vi "Lift_State_Machine.vi"() -> ()   [LabVIEW 2016]
doc: "The state machine for the Lift System.\nDrives the lift forward, then upward, then back, then down to its origin."
uses:
  <vilib>/myRIO/Instrument Drivers/Onboard IO/AI/typedefs/AI Reference.ctl
  <vilib>/myRIO/Common/Instrument Driver Framework/Utilities/typedefs/myRIO Generic Hardware Reference.ctl
  <vilib>/myRIO/Common/Instrument Driver Framework/Utilities/typedefs/Hardware Version Enum.ctl
  <vilib>/myRIO/Common/Instrument Driver Framework/Utilities/typedefs/myRIO v1.0 Reference.ctl
  <vilib>/myRIO/Common/Instrument Driver Framework/Utilities/typedefs/Generic FPGA Reference.ctl
  <vilib>/myRIO/Common/Instrument Driver Framework/myRIO v1.0/AI/typedefs/AI Channels List.ctl
  <vilib>/myRIO/Common/Instrument Driver Framework/myRIO v1.0/AI/typedefs/AI Channels Enum.ctl
  <vilib>/myRIO/Common/Instrument Driver Framework/Utilities/typedefs/Analog Scaling Constants List.ctl
  <vilib>/myRIO/Common/Instrument Driver Framework/Utilities/typedefs/Analog Scaling Constants.ctl
  <vilib>/userdefined/High Color/nirio_resource_hc.ctl
  <vilib>/myRIO/Instrument Drivers/Onboard IO/DIO/typedefs/DIO Reference.ctl
  <vilib>/myRIO/Common/Instrument Driver Framework/myRIO v1.0/DIO/typedefs/DIO Channels List.ctl
  <vilib>/myRIO/Common/Instrument Driver Framework/myRIO v1.0/DIO/typedefs/DIO Channels Enum.ctl
  <vilib>/myRIO/Common/Instrument Driver Framework/Utilities/vis/Is FPGA Ref Available.vi
  <vilib>/myRIO/Common/Instrument Driver Framework/roboRIO v1.0/DIO/vis/roboRIO v1.0 Open DIO.vi
  <vilib>/myRIO/Instrument Drivers/Onboard IO/DIO/vis/Write.vi
  <vilib>/myRIO/Instrument Drivers/Onboard IO/DIO/vis/Read.vi
  <vilib>/myRIO/Common/Instrument Driver Framework/roboRIO v1.0/AI/vis/roboRIO v1.0 Open AI.vi
  <vilib>/myRIO/Instrument Drivers/Onboard IO/AI/vis/Read.vi
  <vilib>/myRIO/Common/Instrument Driver Framework/Utilities/vis/Validate Channels.vi
  <vilib>/myRIO/Common/Instrument Driver Framework/roboRIO v1.0/DIO/vis/roboRIO v1.0 Reserve DIO.vi
  <vilib>/myRIO/Common/Instrument Driver Framework/roboRIO v1.0/AI/vis/roboRIO v1.0 Reserve AI.vi
  <vilib>/myRIO/Common/Instrument Driver Framework/roboRIO v1.0/DIO/vis/roboRIO v1.0 Build MUX Configuration DIO.vi
  <vilib>/myRIO/Common/Instrument Driver Framework/roboRIO v1.0/Resource Manager/vis/roboRIO v1.0 Reserve Channel List.vi
  <vilib>/myRIO/Common/Instrument Driver Framework/roboRIO v1.0/AI/vis/roboRIO v1.0 Build MUX Configuration AI.vi
  <vilib>/myRIO/Common/Instrument Driver Framework/roboRIO v1.0/Resource Manager/vis/roboRIO v1.0 Create Configuration List.vi
  <vilib>/myRIO/Common/Instrument Driver Framework/roboRIO v1.0/Resource Manager/vis/roboRIO v1.0 Reserve Channel.vi
  <vilib>/myRIO/Common/Instrument Driver Framework/roboRIO v1.0/Resource Manager/vis/roboRIO v1.0 Unreserve Channel.vi
  <vilib>/myRIO/Common/Instrument Driver Framework/roboRIO v1.0/Resource Manager/vis/roboRIO v1.0 Build Mutex Name.vi
  GlobalVI.vi
  <vilib>/Utility/VariantDataType/GetNumericInfo.vi
  builds/UnicornMain/UnicornRIO1/ROS for LabVIEW/home/lvuser/natinst/bin/vi.lib/Utility/error.llb/Error Cluster From Error Code.vi
  <vilib>/myRIO/Common/Instrument Driver Framework/roboRIO v1.0/roboRIO v1.0 Open.vi
  <vilib>/myRIO/Common/Instrument Driver Framework/roboRIO v1.0/AI/vis/roboRIO v1.0 Get Scaling Constants AI.vi
  <vilib>/myRIO/Common/Instrument Driver Framework/Utilities/vis/IO Manager.vi
  <vilib>/myRIO/Common/Instrument Driver Framework/Utilities/vis/Configuration Manager.vi
  <vilib>/myRIO/Common/Instrument Driver Framework/myRIO v1.0/myRIO v1.0 Close.vi
  <vilib>/myRIO/Common/Instrument Driver Framework/roboRIO v1.0/AI/vis/roboRIO v1.0 Read AI.vi
  <vilib>/myRIO/Common/Instrument Driver Framework/roboRIO v1.0/Resource Manager/vis/roboRIO v1.0 Configure IO.vi
  <vilib>/myRIO/Common/Instrument Driver Framework/roboRIO v1.0/DIO/vis/roboRIO v1.0 Read DIO.vi
  <vilib>/myRIO/Common/Instrument Driver Framework/roboRIO v1.0/DIO/vis/roboRIO v1.0 Write DIO.vi
  <vilib>/myRIO/Express VI/Onboard IO/AI/AI Express VI.xnode
  <vilib>/myRIO/Instrument Drivers/Onboard IO/AI/vis/myRIO AI Open.xnode
  <vilib>/myRIO/Express VI/Onboard IO/DI/DI Express VI.xnode
  <vilib>/myRIO/Instrument Drivers/Onboard IO/DIO/vis/myRIO DIO Open.xnode
  <vilib>/myRIO/Express VI/Onboard IO/DO/DO Express VI.xnode
  <vilib>/myRIO/Express VI/Onboard Devices/LED/LED Express VI.xnode
  <vilib>/myRIO/Instrument Drivers/Onboard IO/DIO/DIO.lvlib
  <vilib>/myRIO/Instrument Drivers/Onboard IO/AI/AI.lvlib
panel:
  out "B/DIO10 (Pin 31)":bool
  out "B/DIO7 (Pin 25)":bool
  out "PickingRoutine":i32
  out "TrashCanOn 2":bool
  out "Emergency stop sensor":dbl
  out "VIN Gauge":dbl(knob) scale=0.0..4.0
  out "B/DIO10 (Pin 31) - Sensor 5\nBackwards":bool
  out "B/DIO10 (Pin 31) - Sensor 5\nBackwards":bool
  out "liftState":i32
  out "timerCount":u32
  out "timeoutError":bool
  out "timeoutCounter":u32
  out "B/DIO7 (Pin 25) - Sensor2 - Down":bool
  out "B/DIO8 (Pin 27) - Sensor 3 - Up":bool
  out "B/DIO9 (Pin 29) - Sensor 4 - Forward":bool
  out "B/DIO7 (Pin 25) - Sensor 2 - Down":bool
  out "B/DIO9 (Pin 29) - Sensor4 - Forward":bool
  out "B/DIO8 (Pin 27) - Sensor3 - Up":bool
  out "TrashCanOn":bool
  out "DIO/DIO4 (Pin 4) - Emergency stop":bool
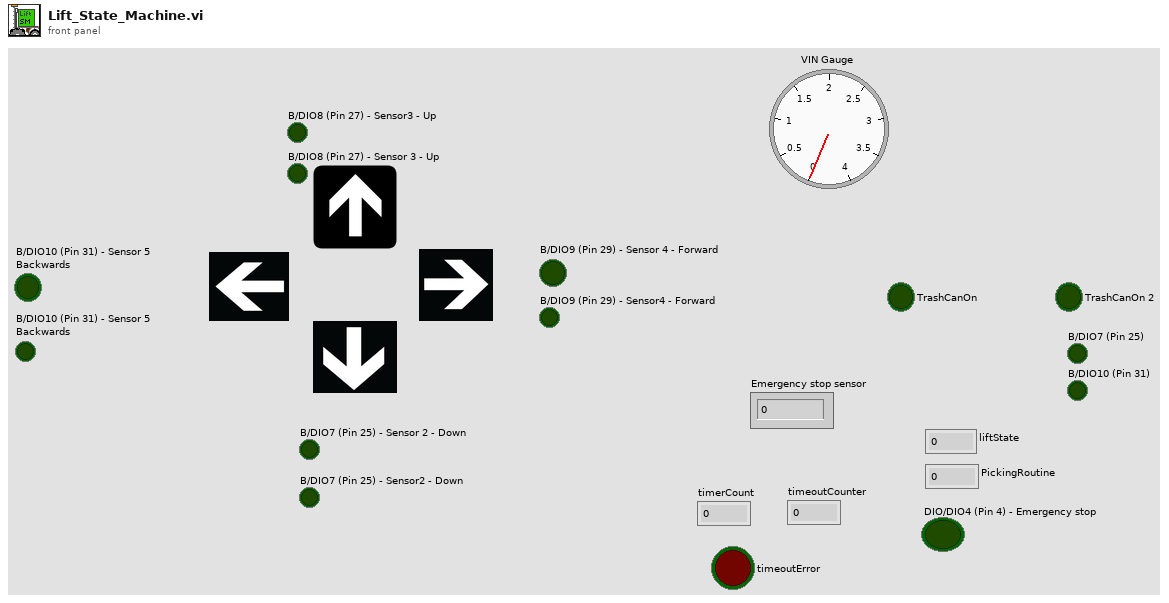
[diagram p1: front panel]
types:
  T1 = typedef "DIO.lvlib/DIO Reference.ctl" = cluster{"myRIO Reference":T2, "DIO Channels List":T6}
  T2 = typedef "myRIO Generic Hardware Reference.ctl" = cluster{"myRIO Model":T3, "myRIO Hardware Reference":T4}
  T3 = typedef "Hardware Version Enum.ctl" = enum16{"Unknown", "myRIO-1900", "myRIO-1950", "roboRIO", "NI ELVIS RIO CM"}
  T4 = typedef "myRIO v1.0 Reference.ctl" = cluster{"Generic FPGA Reference":T5, "Allow multiple opens":bool}
  T5 = typedef "Generic FPGA Reference.ctl" = refnum<k20>
  T6 = typedef "DIO Channels List.ctl" = T7[]
  T7 = typedef "DIO Channels Enum.ctl" = enum16{"Not Connected", "C/DIO0", "C/DIO1", "C/DIO2", "C/DIO3", "C/DIO4", "C/DIO5", "C/DIO6", "C/DIO7", "A/DIO0", "A/DIO1", "A/DIO2", "A/DIO3", "A/DIO4", "A/DIO5", "A/DIO6", "A/DIO7", "A/DIO8", "A/DIO9", "A/DIO10", "A/DIO11", "A/DIO12", "A/DIO13", "A/DIO14", "A/DIO15", "B/DIO0", "B/DIO1", "B/DIO2", "B/DIO3", "B/DIO4", "B/DIO5", "B/DIO6", "B/DIO7", "B/DIO8", "B/DIO9", "B/DIO10", "B/DIO11", "B/DIO12", "B/DIO13", "B/DIO14", "B/DIO15", "LED0", "LED1", "LED2", "LED3", "Button0", "DIO/DIO0", "DIO/DIO1", "DIO/DIO2", "DIO/DIO3", "DIO/DIO4", "DIO/DIO5", "DIO/DIO6", "DIO/DIO7", "DIO/DIO8", "DIO/DIO9", "SPI/CS0", "SPI/CS1", "SPI/CS2", "SPI/CS3", "LED RADIO (Green)", "LED RADIO (Red)", "LED COMM (Green)", "LED COMM (Red)", "LED MODE (Green)", "LED MODE (Red)"}
  T8 = typedef "nirio_resource_hc.ctl" = tag
  T9 = typedef "AI.lvlib/AI Reference.ctl" = cluster{"myRIO Reference":T2, "AI Channels List":T10, "AI Scaling Constants List":T12}
  T10 = typedef "AI Channels List.ctl" = T11[]
  T11 = typedef "AI Channels Enum.ctl" = enum16{"Not Connected", "AudioIn/Left", "AudioIn/Right", "C/AI0", "C/AI1", "A/AI0", "A/AI1", "A/AI2", "A/AI3", "B/AI0", "B/AI1", "B/AI2", "B/AI3", "AI/AI0", "AI/AI1", "AI/AI2", "AI/AI3"}
  T12 = typedef "Analog Scaling Constants List.ctl" = T13[]
  T13 = typedef "Analog Scaling Constants.ctl" = cluster{"LSB Weight (Volts)":dbl, "Offset (Volts)":dbl, "Signed?":bool}
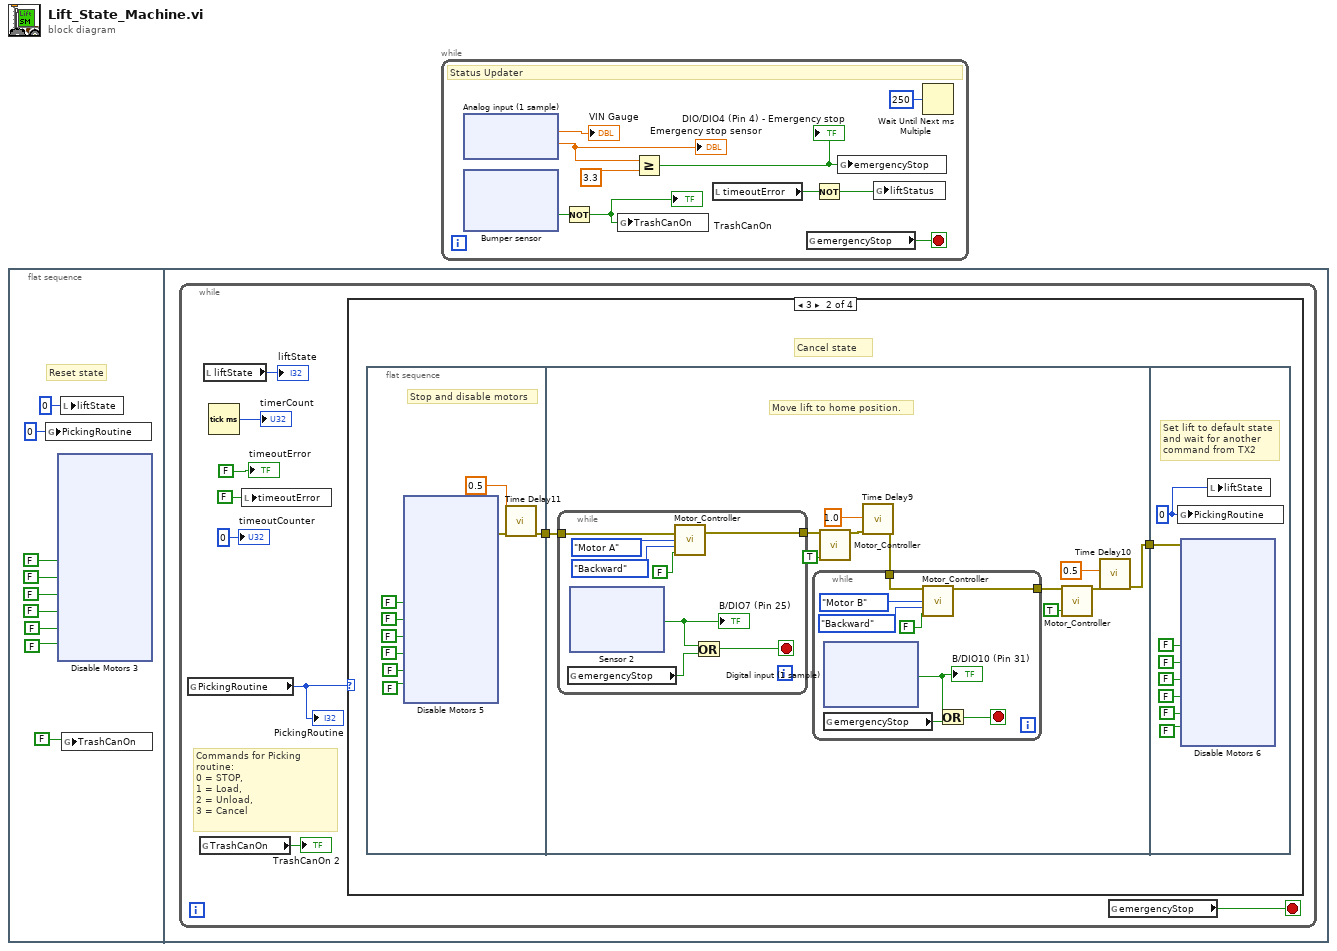
[diagram p0: block diagram]
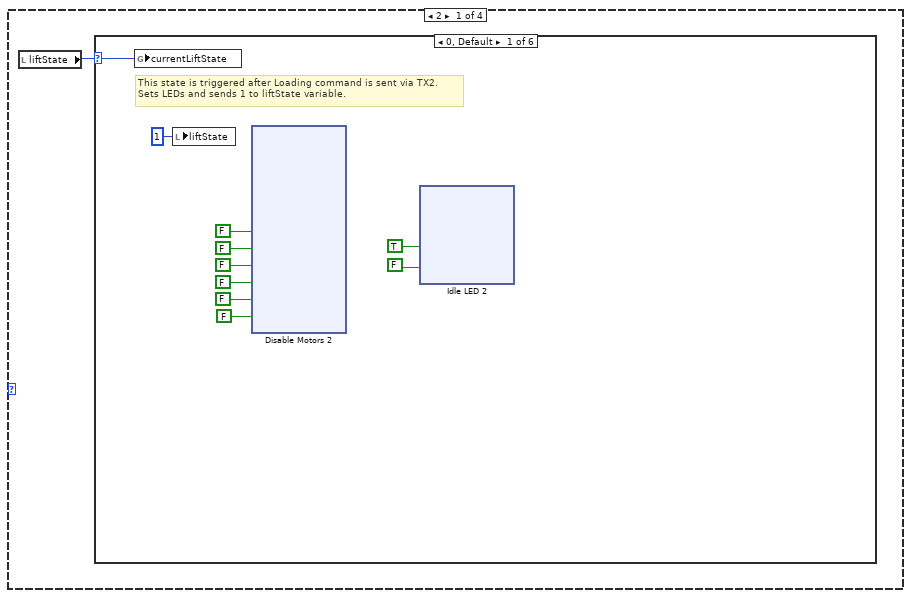
[diagram p2: hidden frame]
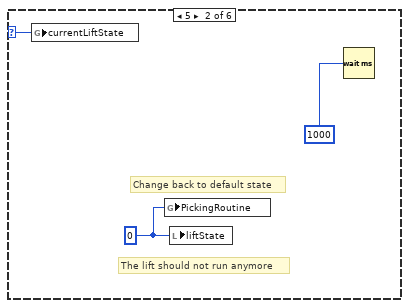
[diagram p3: hidden frame]
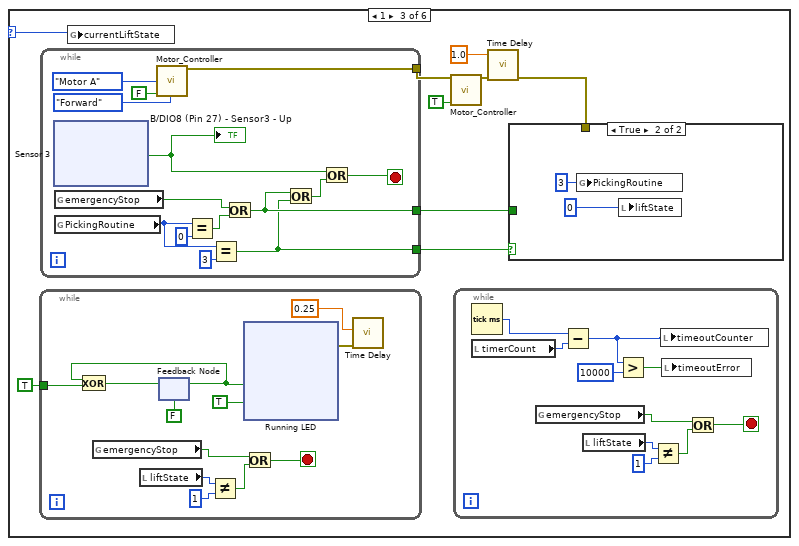
[diagram p4: hidden frame]
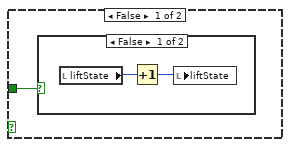
[diagram p5: hidden frame]
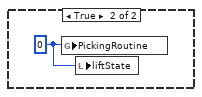
[diagram p6: hidden frame]
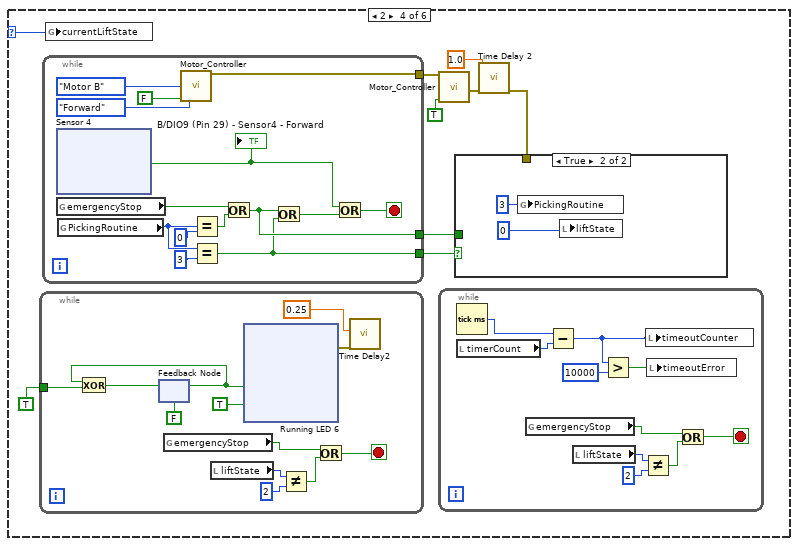
[diagram p7: hidden frame]
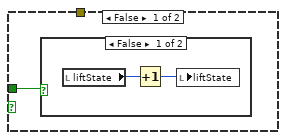
[diagram p8: hidden frame]
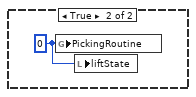
[diagram p9: hidden frame]
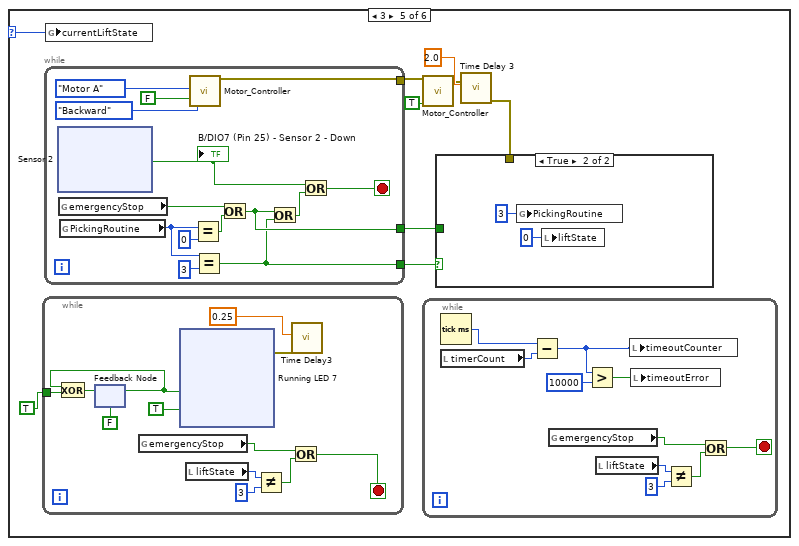
[diagram p10: hidden frame]
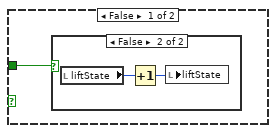
[diagram p11: hidden frame]
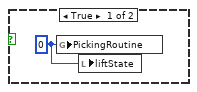
[diagram p12: hidden frame]
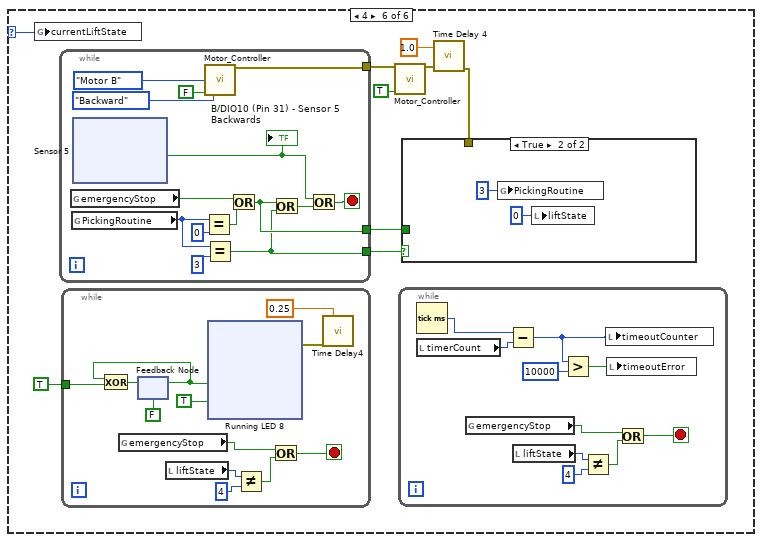
[diagram p13: hidden frame]
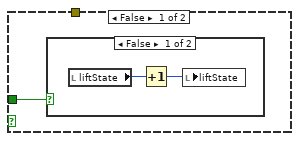
[diagram p14: hidden frame]
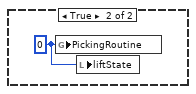
[diagram p15: hidden frame]
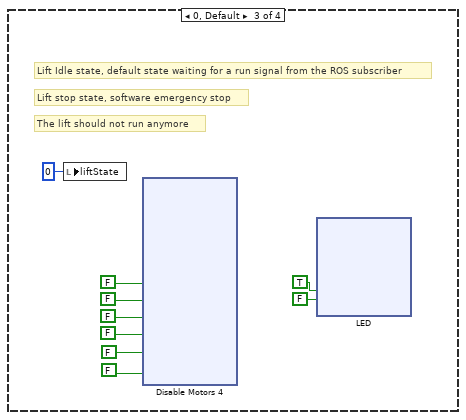
[diagram p16: hidden frame]
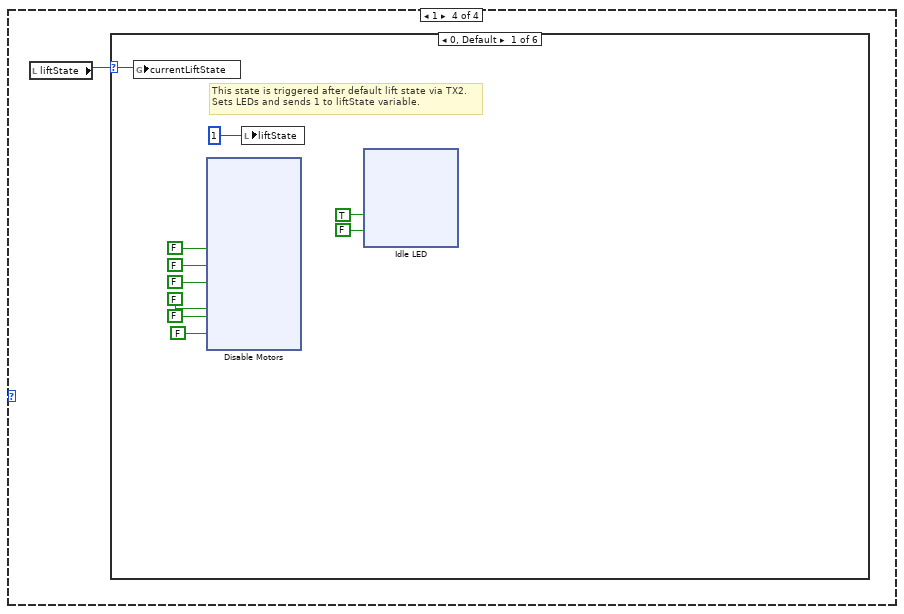
[diagram p17: hidden frame]
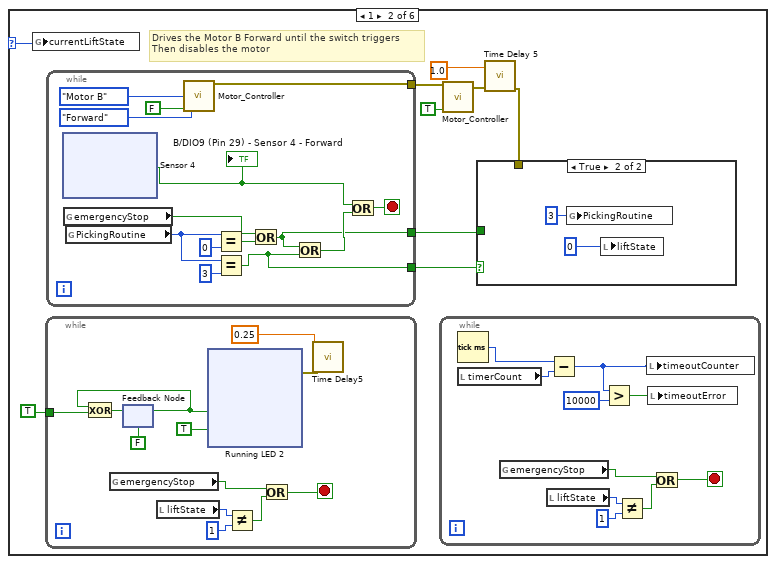
[diagram p18: hidden frame]
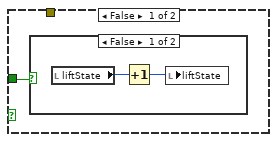
[diagram p19: hidden frame]
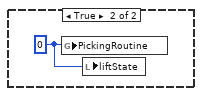
[diagram p20: hidden frame]
diagram:
  n1 = flat-sequence {
    frame #0 {
      # "Reset state"
      n2 = global write "GlobalVI.vi" "PickingRoutine"(0 ("PickingRoutine")) -> ()
      n3 = xnode "Disable Motors 3"("IN1 (B/DIO1 (Pin 13))"=FALSE ("IN2 (B/DIO1 (Pin 13))"), "IN2 (B/DIO2 (Pin 15))"=FALSE ("IN3 (B/DIO2 (Pin 15))"), "IN3 (B/DIO4 (Pin 19))"=FALSE ("IN4 (B/DIO3 (Pin 17))"), "IN4 (B/DIO3 (Pin 17))"=FALSE ("ENABLE A (B/DIO13 (Pin 26))"), "ENABLE A (B/DIO0 (Pin 11))"=FALSE ("ENABLE B (B/DIO8 (Pin 27))"), "ENABLE B (B/DIO5 (Pin 21))"=FALSE ("ENABLE B (B/DIO8 (Pin 27))")) -> ()  [unwired: 1 in, 1 out]
      n4 = local write "liftState"(0 ("liftState")) -> ()
      n5 = global write "GlobalVI.vi" "TrashCanOn"(FALSE) -> ()
    }
    frame #1 {
      n6 = while {
        stop <- w57 stop-if-true
        # "Commands for Picking routine: \n0 = STOP,  \n1 = Load, \n2 = Unload, \n3 = Cancel"
        n7 = global read "GlobalVI.vi" "PickingRoutine"() -> (w50:i32)
        "PickingRoutine" <- w50
        n8 = global read "GlobalVI.vi" "TrashCanOn"() -> (→"TrashCanOn 2":bool)
        n9 = local read "liftState"() -> (→"liftState":i32)
        n10 = Tick Count (ms)() -> (millisecond timer value=→"timerCount":u32)
        n11 = local write "timeoutError"(FALSE ("timeoutError")) -> ()
        n12 = case shown="3" w50 {
          frame 2 {
            n13 = local read "liftState"() -> (w58:i32)
            n14 = case shown="0, Default" w58 {
              selector: w58 -> [w65 w147 w156 w273 w395 w517]
              frame 0, Default {
                # "This state is triggered after Loading command is sent via TX2. \nSets LEDs and sends 1 to liftState variable."
                n15 = global write "GlobalVI.vi" "currentLiftState"(w65) -> ()
                n16 = local write "liftState"(1 ("liftState")) -> ()
                n17 = xnode "Disable Motors 2"("IN1 (B/DIO1 (Pin 13))"=FALSE ("IN1 (B/DIO0 (Pin 11))"), "IN2 (B/DIO2 (Pin 15))"=FALSE ("IN2 (B/DIO1 (Pin 13))"), "IN3 (B/DIO4 (Pin 19))"=FALSE ("IN3 (B/DIO2 (Pin 15))"), "IN4 (B/DIO3 (Pin 17))"=FALSE, "ENABLE A (B/DIO0 (Pin 11))"=FALSE ("ENABLE A (B/DIO13 (Pin 26))"), "ENABLE B (B/DIO5 (Pin 21))"=FALSE ("ENABLE B (B/DIO8 (Pin 27))")) -> ()  [unwired: 1 in, 1 out]
                n18 = xnode "Idle LED 2"("CommG"=TRUE, "CommR"=FALSE ("CommG")) -> ()  [unwired: 1 in, 1 out]
              }
              frame 5 {
                w145 = 0 ("liftState")
                # "The lift should not run anymore"
                # "Change back to default state"
                n19 = global write "GlobalVI.vi" "currentLiftState"(w147) -> ()
                n20 = global write "GlobalVI.vi" "PickingRoutine"(w145) -> ()
                n21 = local write "liftState"(w145) -> ()
                n22 = Wait (ms)(milliseconds to wait=u32 1000) -> ()  [unwired: 1 out]
              }
              frame 1 {
                n23 = while {
                  tunnel: TRUE ("COMM (Red)") -> [w184]
                  stop <- w174 stop-if-true
                  n24 = global read "GlobalVI.vi" "emergencyStop"() -> (w175:bool)
                  n25 = local read "liftState"() -> (w177:i32)
                  n26 = feedback #1(FALSE) -> (w182:bool)
                  n27 = Exclusive Or(1:w184, 2:w182) -> (0:w183:bool)
                  n28 = feedback-in #1(w183) -> ()
                  n29 = Not Equal?(x=w177, y=1 ("liftState")) -> (x != y?=w176:bool)
                  n30 = xnode "Running LED"("CommG"=w182, "CommR"=TRUE) -> ("error out"=w179:errorcluster)  [unwired: 1 in]
                  n31 = Or(x=w175, y=w176) -> (x .or. y?=w174:bool)
                  n32 = call "Time Delay"("error in (no error)"=w179, "Delay Time (s)"=0.25) -> ()  [unwired: 9 in, 1 out]
                }
                n33 = while {
                  tunnel: [w233] -> w151
                  tunnel: [w224] -> w148
                  tunnel: [w221] -> w149
                  stop <- w234 stop-if-true
                  n34 = xnode "Sensor 3"() -> ("B/DIO8 (Pin 27)"=w229:bool)  [unwired: 1 in, 1 out]
                  "B/DIO8 (Pin 27) - Sensor3 - Up" <- w229
                  n35 = global read "GlobalVI.vi" "emergencyStop"() -> (w226:bool)
                  n36 = global read "GlobalVI.vi" "PickingRoutine"() -> (w223:i32)
                  n37 = call "Motor_Controller.vi"("motorSelect"=enum16{"Motor A", "Motor B"}."Motor A", "direction"=enum16{"Forward", "Backward"}."Forward", "stopMotors"=FALSE) -> ("error out"=w233:errorcluster)  [unwired: 12 in]
                  n38 = Equal?(x=w223, y=0) -> (x = y?=w227:bool)
                  n39 = Equal?(x=w223, y=3) -> (x = y?=w221:bool)
                  n40 = Or(x=w226, y=w227) -> (x .or. y?=w224:bool)
                  n41 = Or(x=w224, y=w221) -> (x .or. y?=w222:bool)
                  n42 = Or(x=w229, y=w222) -> (x .or. y?=w234:bool)
                }
                n43 = global write "GlobalVI.vi" "currentLiftState"(w156) -> ()
                n44 = call "Motor_Controller.vi"("error in (no error)"=w151, "stopMotors"=TRUE) -> ("error out"=w152:errorcluster)  [unwired: 13 in]
                n45 = while {
                  stop <- w166 stop-if-true
                  n46 = Tick Count (ms)() -> (millisecond timer value=w172:u32)
                  n47 = local read "timerCount"() -> (w171:u32)
                  n48 = global read "GlobalVI.vi" "emergencyStop"() -> (w170:bool)
                  n49 = Subtract(x=w172, y=w171) -> (x-y=w163:u32)
                  n50 = local read "liftState"() -> (w168:i32)
                  n51 = Greater?(x=w163, y=u32 10000) -> (0:w164:bool)
                  n52 = Not Equal?(x=w168, y=1 ("liftState")) -> (x != y?=w169:bool)
                  n53 = local write "timeoutCounter"(w163) -> ()
                  n54 = local write "timeoutError"(w164) -> ()
                  n55 = Or(x=w170, y=w169) -> (x .or. y?=w166:bool)
                }
                n56 = call "Time Delay"("error in (no error)"=w152, "Delay Time (s)"=1.0) -> ("error out"=w150:errorcluster)  [unwired: 9 in]
                n57 = case shown="True" w149 {
                  tunnel: w150 -> [_ _]
                  tunnel: w148 -> [w157 _]
                  frame False {
                    n58 = case shown="False" w157 {
                      frame False {
                        n59 = local read "liftState"() -> (w159:i32)
                        n60 = Increment(x=w159) -> (x+1=w158:i32)
                        n61 = local write "liftState"(w158) -> ()
                      }
                      frame True {
                        w160 = 0 ("liftState")
                        n62 = global write "GlobalVI.vi" "PickingRoutine"(w160) -> ()
                        n63 = local write "liftState"(w160) -> ()
                      }
                    }
                  }
                  frame True {
                    n64 = global write "GlobalVI.vi" "PickingRoutine"(3 ("PickingRoutine")) -> ()
                    n65 = local write "liftState"(0 ("liftState")) -> ()
                  }
                }
              }
              frame 2 {
                n66 = while {
                  tunnel: TRUE ("COMM (Red)") -> [w306]
                  stop <- w296 stop-if-true
                  n67 = feedback #2(FALSE) -> (w304:bool)
                  n68 = Exclusive Or(1:w306, 2:w304) -> (0:w305:bool)
                  n69 = feedback-in #2(w305) -> ()
                  n70 = global read "GlobalVI.vi" "emergencyStop"() -> (w297:bool)
                  n71 = local read "liftState"() -> (w299:i32)
                  n72 = xnode "Running LED 6"("CommG"=w304, "CommR"=TRUE) -> ("error out"=w301:errorcluster)  [unwired: 1 in]
                  n73 = Not Equal?(x=w299, y=2 ("liftState")) -> (x != y?=w298:bool)
                  n74 = Or(x=w297, y=w298) -> (x .or. y?=w296:bool)
                  n75 = call "Time Delay2"("error in (no error)"=w301, "Delay Time (s)"=0.25) -> ()  [unwired: 9 in, 1 out]
                }
                n76 = while {
                  tunnel: [w355] -> w274
                  tunnel: [w345] -> w271
                  tunnel: [w343] -> w272
                  stop <- w356 stop-if-true
                  n77 = xnode "Sensor 4"() -> ("B/DIO9 (Pin 29)"=w351:bool)  [unwired: 1 in, 1 out]
                  "B/DIO9 (Pin 29) - Sensor4 - Forward" <- w351
                  n78 = global read "GlobalVI.vi" "emergencyStop"() -> (w348:bool)
                  n79 = global read "GlobalVI.vi" "PickingRoutine"() -> (w346:i32)
                  n80 = call "Motor_Controller.vi"("motorSelect"=enum16{"Motor A", "Motor B"}."Motor B", "direction"=enum16{"Forward", "Backward"}."Forward", "stopMotors"=FALSE) -> ("error out"=w355:errorcluster)  [unwired: 12 in]
                  n81 = Equal?(x=w346, y=0) -> (x = y?=w349:bool)
                  n82 = Equal?(x=w346, y=3) -> (x = y?=w343:bool)
                  n83 = Or(x=w348, y=w349) -> (x .or. y?=w345:bool)
                  n84 = Or(x=w345, y=w343) -> (x .or. y?=w344:bool)
                  n85 = Or(x=w351, y=w344) -> (x .or. y?=w356:bool)
                }
                n86 = global write "GlobalVI.vi" "currentLiftState"(w273) -> ()
                n87 = call "Motor_Controller.vi"("error in (no error)"=w274, "stopMotors"=TRUE) -> ("error out"=w275:errorcluster)  [unwired: 13 in]
                n88 = while {
                  stop <- w288 stop-if-true
                  n89 = Tick Count (ms)() -> (millisecond timer value=w294:u32)
                  n90 = local read "timerCount"() -> (w293:u32)
                  n91 = global read "GlobalVI.vi" "emergencyStop"() -> (w292:bool)
                  n92 = Subtract(x=w294, y=w293) -> (x-y=w285:u32)
                  n93 = local read "liftState"() -> (w290:i32)
                  n94 = Greater?(x=w285, y=u32 10000) -> (0:w286:bool)
                  n95 = Not Equal?(x=w290, y=2 ("liftState")) -> (x != y?=w291:bool)
                  n96 = local write "timeoutCounter"(w285) -> ()
                  n97 = local write "timeoutError"(w286) -> ()
                  n98 = Or(x=w292, y=w291) -> (x .or. y?=w288:bool)
                }
                n99 = call "Time Delay 2"("error in (no error)"=w275, "Delay Time (s)"=1.0) -> ("error out"=w270:errorcluster)  [unwired: 9 in]
                n100 = case shown="True" w272 {
                  tunnel: w271 -> [w279 _]
                  tunnel: w270 -> [_ _]
                  frame False {
                    n101 = case shown="False" w279 {
                      frame False {
                        n102 = local read "liftState"() -> (w281:i32)
                        n103 = Increment(x=w281) -> (x+1=w280:i32)
                        n104 = local write "liftState"(w280) -> ()
                      }
                      frame True {
                        w282 = 0 ("PickingRoutine")
                        n105 = global write "GlobalVI.vi" "PickingRoutine"(w282) -> ()
                        n106 = local write "liftState"(w282) -> ()
                      }
                    }
                  }
                  frame True {
                    n107 = global write "GlobalVI.vi" "PickingRoutine"(3 ("PickingRoutine")) -> ()
                    n108 = local write "liftState"(0 ("liftState")) -> ()
                  }
                }
              }
              frame 3 {
                n109 = while {
                  tunnel: TRUE ("COMM (Red)") -> [w428]
                  stop <- w418 stop-if-true
                  n110 = feedback #3(FALSE) -> (w426:bool)
                  n111 = Exclusive Or(1:w428, 2:w426) -> (0:w427:bool)
                  n112 = feedback-in #3(w427) -> ()
                  n113 = global read "GlobalVI.vi" "emergencyStop"() -> (w419:bool)
                  n114 = xnode "Running LED 7"("CommG"=w426, "CommR"=TRUE) -> ("error out"=w423:errorcluster)  [unwired: 1 in]
                  n115 = local read "liftState"() -> (w421:i32)
                  n116 = Not Equal?(x=w421, y=3 ("liftState")) -> (x != y?=w420:bool)
                  n117 = Or(x=w419, y=w420) -> (x .or. y?=w418:bool)
                  n118 = call "Time Delay3"("error in (no error)"=w423, "Delay Time (s)"=0.25) -> ()  [unwired: 9 in, 1 out]
                }
                n119 = while {
                  tunnel: [w478] -> w396
                  tunnel: [w466] -> w393
                  tunnel: [w465] -> w392
                  stop <- w473 stop-if-true
                  n120 = xnode "Sensor 2"() -> ("Downwards (B/DIO7 (Pin 25))"=w474:bool)  [unwired: 1 in, 1 out]
                  "B/DIO7 (Pin 25) - Sensor 2 - Down" <- w474
                  n121 = global read "GlobalVI.vi" "emergencyStop"() -> (w471:bool)
                  n122 = global read "GlobalVI.vi" "PickingRoutine"() -> (w468:i32)
                  n123 = call "Motor_Controller.vi"("motorSelect"=enum16{"Motor A", "Motor B"}."Motor A", "direction"=enum16{"Forward", "Backward"}."Backward", "stopMotors"=FALSE) -> ("error out"=w478:errorcluster)  [unwired: 12 in]
                  n124 = Equal?(x=w468, y=0) -> (x = y?=w470:bool)
                  n125 = Equal?(x=w468, y=3) -> (x = y?=w465:bool)
                  n126 = Or(x=w471, y=w470) -> (x .or. y?=w466:bool)
                  n127 = Or(x=w466, y=w465) -> (x .or. y?=w467:bool)
                  n128 = Or(x=w474, y=w467) -> (x .or. y?=w473:bool)
                }
                n129 = global write "GlobalVI.vi" "currentLiftState"(w395) -> ()
                n130 = call "Motor_Controller.vi"("error in (no error)"=w396, "stopMotors"=TRUE) -> ("error out"=w397:errorcluster)  [unwired: 13 in]
                n131 = while {
                  stop <- w410 stop-if-true
                  n132 = Tick Count (ms)() -> (millisecond timer value=w416:u32)
                  n133 = local read "timerCount"() -> (w415:u32)
                  n134 = Subtract(x=w416, y=w415) -> (x-y=w407:u32)
                  n135 = global read "GlobalVI.vi" "emergencyStop"() -> (w414:bool)
                  n136 = Greater?(x=w407, y=u32 10000) -> (0:w408:bool)
                  n137 = local read "liftState"() -> (w412:i32)
                  n138 = local write "timeoutCounter"(w407) -> ()
                  n139 = local write "timeoutError"(w408) -> ()
                  n140 = Not Equal?(x=w412, y=3 ("liftState")) -> (x != y?=w413:bool)
                  n141 = Or(x=w414, y=w413) -> (x .or. y?=w410:bool)
                }
                n142 = call "Time Delay 3"("error in (no error)"=w397, "Delay Time (s)"=2.0) -> ("error out"=w394:errorcluster)  [unwired: 9 in]
                n143 = case shown="True" w392 {
                  tunnel: w394 -> [_ _]
                  tunnel: w393 -> [w401 _]
                  frame False {
                    n144 = case shown="False" w401 {
                      frame True {
                        w402 = 0 ("PickingRoutine")
                        n145 = global write "GlobalVI.vi" "PickingRoutine"(w402) -> ()
                        n146 = local write "liftState"(w402) -> ()
                      }
                      frame False {
                        n147 = local read "liftState"() -> (w403:i32)
                        n148 = Increment(x=w403) -> (x+1=w404:i32)
                        n149 = local write "liftState"(w404) -> ()
                      }
                    }
                  }
                  frame True {
                    n150 = global write "GlobalVI.vi" "PickingRoutine"(3 ("PickingRoutine")) -> ()
                    n151 = local write "liftState"(0 ("liftState")) -> ()
                  }
                }
              }
              frame 4 {
                n152 = global write "GlobalVI.vi" "currentLiftState"(w517) -> ()
                n153 = while {
                  tunnel: [w599] -> w518
                  tunnel: [w590] -> w515
                  tunnel: [w587] -> w516
                  stop <- w600 stop-if-true
                  n154 = global read "GlobalVI.vi" "emergencyStop"() -> (w592:bool)
                  n155 = global read "GlobalVI.vi" "PickingRoutine"() -> (w588:i32)
                  n156 = xnode "Sensor 5"() -> ("B/DIO10 (Pin 31)"=w595:bool)  [unwired: 1 in, 1 out]
                  "B/DIO10 (Pin 31) - Sensor 5\nBackwards" <- w595
                  n157 = Equal?(x=w588, y=0) -> (x = y?=w593:bool)
                  n158 = call "Motor_Controller.vi"("motorSelect"=enum16{"Motor A", "Motor B"}."Motor B", "direction"=enum16{"Forward", "Backward"}."Backward", "stopMotors"=FALSE) -> ("error out"=w599:errorcluster)  [unwired: 12 in]
                  n159 = Equal?(x=w588, y=3) -> (x = y?=w587:bool)
                  n160 = Or(x=w592, y=w593) -> (x .or. y?=w590:bool)
                  n161 = Or(x=w590, y=w587) -> (x .or. y?=w589:bool)
                  n162 = Or(x=w595, y=w589) -> (x .or. y?=w600:bool)
                }
                n163 = while {
                  tunnel: TRUE ("COMM (Red)") -> [w550]
                  stop <- w540 stop-if-true
                  n164 = global read "GlobalVI.vi" "emergencyStop"() -> (w541:bool)
                  n165 = feedback #4(FALSE) -> (w548:bool)
                  n166 = Exclusive Or(1:w550, 2:w548) -> (0:w549:bool)
                  n167 = feedback-in #4(w549) -> ()
                  n168 = local read "liftState"() -> (w543:i32)
                  n169 = xnode "Running LED 8"("CommG"=w548, "CommR"=TRUE) -> ("error out"=w545:errorcluster)  [unwired: 1 in]
                  n170 = Not Equal?(x=w543, y=4 ("liftState")) -> (x != y?=w542:bool)
                  n171 = Or(x=w541, y=w542) -> (x .or. y?=w540:bool)
                  n172 = call "Time Delay4"("error in (no error)"=w545, "Delay Time (s)"=0.25) -> ()  [unwired: 9 in, 1 out]
                }
                n173 = call "Motor_Controller.vi"("error in (no error)"=w518, "stopMotors"=TRUE) -> ("error out"=w519:errorcluster)  [unwired: 13 in]
                n174 = while {
                  stop <- w532 stop-if-true
                  n175 = Tick Count (ms)() -> (millisecond timer value=w538:u32)
                  n176 = local read "timerCount"() -> (w537:u32)
                  n177 = global read "GlobalVI.vi" "emergencyStop"() -> (w536:bool)
                  n178 = Subtract(x=w538, y=w537) -> (x-y=w529:u32)
                  n179 = local read "liftState"() -> (w534:i32)
                  n180 = Greater?(x=w529, y=u32 10000) -> (0:w530:bool)
                  n181 = Not Equal?(x=w534, y=4 ("liftState")) -> (x != y?=w535:bool)
                  n182 = local write "timeoutCounter"(w529) -> ()
                  n183 = local write "timeoutError"(w530) -> ()
                  n184 = Or(x=w536, y=w535) -> (x .or. y?=w532:bool)
                }
                n185 = call "Time Delay 4"("error in (no error)"=w519, "Delay Time (s)"=1.0) -> ("error out"=w514:errorcluster)  [unwired: 9 in]
                n186 = case shown="True" w516 {
                  tunnel: w515 -> [w523 _]
                  tunnel: w514 -> [_ _]
                  frame False {
                    n187 = case shown="False" w523 {
                      frame False {
                        n188 = local read "liftState"() -> (w525:i32)
                        n189 = Increment(x=w525) -> (x+1=w524:i32)
                        n190 = local write "liftState"(w524) -> ()
                      }
                      frame True {
                        w526 = 0 ("PickingRoutine")
                        n191 = global write "GlobalVI.vi" "PickingRoutine"(w526) -> ()
                        n192 = local write "liftState"(w526) -> ()
                      }
                    }
                  }
                  frame True {
                    n193 = global write "GlobalVI.vi" "PickingRoutine"(3 ("PickingRoutine")) -> ()
                    n194 = local write "liftState"(0 ("liftState")) -> ()
                  }
                }
              }
            }
          }
          frame 3 {
            # "Cancel state"
            n195 = flat-sequence {
              tunnel: [w639] -> w636
              tunnel: [w688] -> w637
              tunnel: w636 -> [w687]
              tunnel: w637 -> [w785]
              frame #0 {
                # "Stop and disable motors"
                n196 = xnode "Disable Motors 5"("IN1 (B/DIO1 (Pin 13))"=FALSE ("IN2 (B/DIO1 (Pin 13))"), "IN2 (B/DIO2 (Pin 15))"=FALSE ("IN3 (B/DIO2 (Pin 15))"), "IN3 (B/DIO4 (Pin 19))"=FALSE ("IN4 (B/DIO3 (Pin 17))"), "IN4 (B/DIO3 (Pin 17))"=FALSE ("ENABLE A (B/DIO13 (Pin 26))"), "ENABLE A (B/DIO0 (Pin 11))"=FALSE ("ENABLE B (B/DIO8 (Pin 27))"), "ENABLE B (B/DIO5 (Pin 21))"=FALSE ("ENABLE B (B/DIO8 (Pin 27))")) -> ("error out"=w640:errorcluster)  [unwired: 1 in]
                n197 = call "Time Delay11"("error in (no error)"=w640, "Delay Time (s)"=0.5) -> ("error out"=w639:errorcluster)  [unwired: 9 in]
              }
              frame #1 {
                # "Move lift to home position."
                n198 = while {
                  tunnel: [w742] -> w696
                  tunnel: w687 -> [w741]
                  stop <- w743 stop-if-true
                  n199 = global read "GlobalVI.vi" "emergencyStop"() -> (w745:bool)
                  n200 = xnode "Sensor 2"() -> ("B/DIO7 (Pin 25)"=w744:bool)  [unwired: 1 in, 1 out]
                  "B/DIO7 (Pin 25)" <- w744
                  n201 = call "Motor_Controller.vi"("error in (no error)"=w741, "motorSelect"=enum16{"Motor A", "Motor B"}."Motor A", "direction"=enum16{"Forward", "Backward"}."Backward", "stopMotors"=FALSE) -> ("error out"=w742:errorcluster)  [unwired: 11 in]
                  n202 = Or(x=w744, y=w745) -> (x .or. y?=w743:bool)
                }
                n203 = call "Motor_Controller.vi"("error in (no error)"=w696, "stopMotors"=TRUE) -> ("error out"=w694:errorcluster)  [unwired: 13 in]
                n204 = call "Time Delay9"("error in (no error)"=w694, "Delay Time (s)"=1.0) -> ("error out"=w693:errorcluster)  [unwired: 9 in]
                n205 = while {
                  tunnel: w693 -> [w702]
                  tunnel: [w698] -> w692
                  stop <- w699 stop-if-true
                  n206 = xnode "Digital input (1 sample)"() -> ("B/DIO10 (Pin 31)"=w700:bool)  [unwired: 1 in, 1 out]
                  "B/DIO10 (Pin 31)" <- w700
                  n207 = global read "GlobalVI.vi" "emergencyStop"() -> (w701:bool)
                  n208 = call "Motor_Controller.vi"("error in (no error)"=w702, "motorSelect"=enum16{"Motor A", "Motor B"}."Motor B", "direction"=enum16{"Forward", "Backward"}."Backward", "stopMotors"=FALSE) -> ("error out"=w698:errorcluster)  [unwired: 11 in]
                  n209 = Or(x=w700, y=w701) -> (x .or. y?=w699:bool)
                }
                n210 = call "Motor_Controller.vi"("error in (no error)"=w692, "stopMotors"=TRUE) -> ("error out"=w690:errorcluster)  [unwired: 13 in]
                n211 = call "Time Delay10"("error in (no error)"=w690, "Delay Time (s)"=0.5) -> ("error out"=w688:errorcluster)  [unwired: 9 in]
              }
              frame #2 {
                w784 = 0 ("PickingRoutine")
                # "Set lift to default state\nand wait for another \ncommand from TX2"
                n212 = global write "GlobalVI.vi" "PickingRoutine"(w784) -> ()
                n213 = xnode "Disable Motors 6"("IN1 (B/DIO1 (Pin 13))"=FALSE ("IN2 (B/DIO1 (Pin 13))"), "IN2 (B/DIO2 (Pin 15))"=FALSE ("IN3 (B/DIO2 (Pin 15))"), "IN3 (B/DIO4 (Pin 19))"=FALSE ("IN4 (B/DIO3 (Pin 17))"), "IN4 (B/DIO3 (Pin 17))"=FALSE ("ENABLE A (B/DIO13 (Pin 26))"), "ENABLE A (B/DIO0 (Pin 11))"=FALSE ("ENABLE B (B/DIO8 (Pin 27))"), "ENABLE B (B/DIO5 (Pin 21))"=FALSE ("ENABLE B (B/DIO8 (Pin 27))"), "error in (no error)"=w785) -> ()  [unwired: 1 out]
                n214 = local write "liftState"(w784) -> ()
              }
            }
          }
          frame 0, Default {
            # "Lift stop state, software emergency stop"
            # "Lift Idle state, default state waiting for a run signal from the ROS subscriber"
            # "The lift should not run anymore"
            n215 = local write "liftState"(0 ("liftState")) -> ()
            n216 = xnode "Disable Motors 4"("IN1 (B/DIO1 (Pin 13))"=FALSE ("IN1 (B/DIO0 (Pin 11))"), "IN2 (B/DIO2 (Pin 15))"=FALSE ("IN2 (B/DIO1 (Pin 13))"), "IN3 (B/DIO4 (Pin 19))"=FALSE ("IN3 (B/DIO2 (Pin 15))"), "IN4 (B/DIO3 (Pin 17))"=FALSE, "ENABLE A (B/DIO0 (Pin 11))"=FALSE ("ENABLE A (B/DIO13 (Pin 26))"), "ENABLE B (B/DIO5 (Pin 21))"=FALSE ("ENABLE B (B/DIO8 (Pin 27))")) -> ()  [unwired: 1 in, 1 out]
            n217 = xnode "LED"("COMM (Green)"=TRUE, "COMM (Red)"=FALSE) -> ()  [unwired: 1 in, 1 out]
          }
          frame 1 {
            n218 = local read "liftState"() -> (w917:i32)
            n219 = case shown="0, Default" w917 {
              selector: w917 -> [w924 w1007 w1130 w1251 w1372 w1492]
              frame 0, Default {
                # "This state is triggered after default lift state via TX2. \nSets LEDs and sends 1 to liftState variable."
                n220 = global write "GlobalVI.vi" "currentLiftState"(w924) -> ()
                n221 = xnode "Disable Motors"("IN1 (B/DIO1 (Pin 13))"=FALSE ("IN1 (B/DIO0 (Pin 11))"), "IN2 (B/DIO2 (Pin 15))"=FALSE ("IN2 (B/DIO1 (Pin 13))"), "IN3 (B/DIO4 (Pin 19))"=FALSE ("IN3 (B/DIO2 (Pin 15))"), "IN4 (B/DIO3 (Pin 17))"=FALSE, "ENABLE A (B/DIO0 (Pin 11))"=FALSE ("ENABLE A (B/DIO13 (Pin 26))"), "ENABLE B (B/DIO5 (Pin 21))"=FALSE ("ENABLE B (B/DIO8 (Pin 27))")) -> ()  [unwired: 1 in, 1 out]
                n222 = local write "liftState"(1 ("liftState")) -> ()
                n223 = xnode "Idle LED"("CommG"=TRUE, "CommR"=FALSE ("CommG")) -> ()  [unwired: 1 in, 1 out]
              }
              frame 1 {
                # "Drives the Motor B Forward until the switch triggers\nThen disables the motor"
                n224 = global write "GlobalVI.vi" "currentLiftState"(w1007) -> ()
                n225 = while {
                  tunnel: TRUE ("COMM (Red)") -> [w1040]
                  stop <- w1030 stop-if-true
                  n226 = global read "GlobalVI.vi" "emergencyStop"() -> (w1031:bool)
                  n227 = feedback #5(FALSE) -> (w1038:bool)
                  n228 = Exclusive Or(1:w1040, 2:w1038) -> (0:w1039:bool)
                  n229 = feedback-in #5(w1039) -> ()
                  n230 = local read "liftState"() -> (w1033:i32)
                  n231 = xnode "Running LED 2"("CommG"=w1038, "CommR"=TRUE) -> ("error out"=w1035:errorcluster)  [unwired: 1 in]
                  n232 = Not Equal?(x=w1033, y=1 ("liftState")) -> (x != y?=w1032:bool)
                  n233 = Or(x=w1031, y=w1032) -> (x .or. y?=w1030:bool)
                  n234 = call "Time Delay5"("error in (no error)"=w1035, "Delay Time (s)"=0.25) -> ()  [unwired: 9 in, 1 out]
                }
                n235 = while {
                  tunnel: [w1089] -> w1008
                  tunnel: [w1078] -> w1005
                  tunnel: [w1077] -> w1006
                  stop <- w1090 stop-if-true
                  n236 = xnode "Sensor 4"() -> ("B/DIO9 (Pin 29)"=w1085:bool)  [unwired: 1 in, 1 out]
                  "B/DIO9 (Pin 29) - Sensor 4 - Forward" <- w1085
                  n237 = global read "GlobalVI.vi" "emergencyStop"() -> (w1083:bool)
                  n238 = global read "GlobalVI.vi" "PickingRoutine"() -> (w1080:i32)
                  n239 = call "Motor_Controller.vi"("motorSelect"=enum16{"Motor A", "Motor B"}."Motor B", "direction"=enum16{"Forward", "Backward"}."Forward", "stopMotors"=FALSE) -> ("error out"=w1089:errorcluster)  [unwired: 12 in]
                  n240 = Equal?(x=w1080, y=0) -> (x = y?=w1082:bool)
                  n241 = Equal?(x=w1080, y=3) -> (x = y?=w1077:bool)
                  n242 = Or(x=w1083, y=w1082) -> (x .or. y?=w1078:bool)
                  n243 = Or(x=w1078, y=w1077) -> (x .or. y?=w1079:bool)
                  n244 = Or(x=w1085, y=w1079) -> (x .or. y?=w1090:bool)
                }
                n245 = while {
                  stop <- w1022 stop-if-true
                  n246 = Tick Count (ms)() -> (millisecond timer value=w1028:u32)
                  n247 = local read "timerCount"() -> (w1027:u32)
                  n248 = global read "GlobalVI.vi" "emergencyStop"() -> (w1026:bool)
                  n249 = local read "liftState"() -> (w1024:i32)
                  n250 = Subtract(x=w1028, y=w1027) -> (x-y=w1019:u32)
                  n251 = Greater?(x=w1019, y=u32 10000) -> (0:w1020:bool)
                  n252 = Not Equal?(x=w1024, y=1 ("liftState")) -> (x != y?=w1025:bool)
                  n253 = local write "timeoutCounter"(w1019) -> ()
                  n254 = local write "timeoutError"(w1020) -> ()
                  n255 = Or(x=w1026, y=w1025) -> (x .or. y?=w1022:bool)
                }
                n256 = call "Motor_Controller.vi"("error in (no error)"=w1008, "stopMotors"=TRUE) -> ("error out"=w1009:errorcluster)  [unwired: 13 in]
                n257 = call "Time Delay 5"("error in (no error)"=w1009, "Delay Time (s)"=1.0) -> ("error out"=w1004:errorcluster)  [unwired: 9 in]
                n258 = case shown="True" w1006 {
                  tunnel: w1005 -> [w1013 _]
                  tunnel: w1004 -> [_ _]
                  frame False {
                    n259 = case shown="False" w1013 {
                      frame False {
                        n260 = local read "liftState"() -> (w1015:i32)
                        n261 = Increment(x=w1015) -> (x+1=w1014:i32)
                        n262 = local write "liftState"(w1014) -> ()
                      }
                      frame True {
                        w1016 = 0 ("liftState")
                        n263 = global write "GlobalVI.vi" "PickingRoutine"(w1016) -> ()
                        n264 = local write "liftState"(w1016) -> ()
                      }
                    }
                  }
                  frame True {
                    n265 = global write "GlobalVI.vi" "PickingRoutine"(3 ("PickingRoutine")) -> ()
                    n266 = local write "liftState"(0 ("liftState")) -> ()
                  }
                }
              }
              frame 2 {
                # "Drives the Motor A Up until the switch triggers\nThen disables the motor"
                n267 = global write "GlobalVI.vi" "currentLiftState"(w1130) -> ()
                n268 = while {
                  tunnel: [w1210] -> w1129
                  tunnel: [w1200] -> w1128
                  tunnel: [w1199] -> w1127
                  stop <- w1207 stop-if-true
                  n269 = global read "GlobalVI.vi" "emergencyStop"() -> (w1206:bool)
                  n270 = xnode "Sensor 3"() -> ("Upwards (B/DIO8 (Pin 27))"=w1208:bool)  [unwired: 1 in, 1 out]
                  "B/DIO8 (Pin 27) - Sensor 3 - Up" <- w1208
                  n271 = global read "GlobalVI.vi" "PickingRoutine"() -> (w1202:i32)
                  n272 = call "Motor_Controller.vi"("motorSelect"=enum16{"Motor A", "Motor B"}."Motor A", "direction"=enum16{"Forward", "Backward"}."Forward", "stopMotors"=FALSE) -> ("error out"=w1210:errorcluster)  [unwired: 12 in]
                  n273 = Equal?(x=w1202, y=0) -> (x = y?=w1205:bool)
                  n274 = Equal?(x=w1202, y=3) -> (x = y?=w1200:bool)
                  n275 = Or(x=w1206, y=w1205) -> (x .or. y?=w1201:bool)
                  n276 = Or(x=w1201, y=w1200) -> (x .or. y?=w1199:bool)
                  n277 = Or(x=w1208, y=w1199) -> (x .or. y?=w1207:bool)
                }
                n278 = while {
                  tunnel: TRUE ("COMM (Red)") -> [w1162]
                  stop <- w1152 stop-if-true
                  n279 = global read "GlobalVI.vi" "emergencyStop"() -> (w1153:bool)
                  n280 = feedback #6(FALSE) -> (w1160:bool)
                  n281 = Exclusive Or(1:w1162, 2:w1160) -> (0:w1161:bool)
                  n282 = feedback-in #6(w1161) -> ()
                  n283 = local read "liftState"() -> (w1155:i32)
                  n284 = xnode "Running LED 3"("CommG"=w1160, "CommR"=TRUE) -> ("error out"=w1157:errorcluster)  [unwired: 1 in]
                  n285 = Not Equal?(x=w1155, y=2 ("liftState")) -> (x != y?=w1154:bool)
                  n286 = Or(x=w1153, y=w1154) -> (x .or. y?=w1152:bool)
                  n287 = call "Time Delay6"("error in (no error)"=w1157, "Delay Time (s)"=0.25) -> ()  [unwired: 9 in, 1 out]
                }
                n288 = while {
                  stop <- w1144 stop-if-true
                  n289 = Tick Count (ms)() -> (millisecond timer value=w1150:u32)
                  n290 = local read "timerCount"() -> (w1149:u32)
                  n291 = global read "GlobalVI.vi" "emergencyStop"() -> (w1148:bool)
                  n292 = local read "liftState"() -> (w1146:i32)
                  n293 = Subtract(x=w1150, y=w1149) -> (x-y=w1141:u32)
                  n294 = Not Equal?(x=w1146, y=2 ("liftState")) -> (x != y?=w1147:bool)
                  n295 = Greater?(x=w1141, y=u32 10000) -> (0:w1142:bool)
                  n296 = local write "timeoutCounter"(w1141) -> ()
                  n297 = local write "timeoutError"(w1142) -> ()
                  n298 = Or(x=w1148, y=w1147) -> (x .or. y?=w1144:bool)
                }
                n299 = call "Motor_Controller.vi"("error in (no error)"=w1129, "stopMotors"=TRUE) -> ("error out"=w1131:errorcluster)  [unwired: 13 in]
                n300 = call "Time Delay 6"("error in (no error)"=w1131, "Delay Time (s)"=2.0) -> ("error out"=w1126:errorcluster)  [unwired: 9 in]
                n301 = case shown="True" w1128 {
                  tunnel: w1127 -> [w1135 _]
                  tunnel: w1126 -> [_ _]
                  frame False {
                    n302 = case shown="False" w1135 {
                      frame False {
                        n303 = local read "liftState"() -> (w1137:i32)
                        n304 = Increment(x=w1137) -> (x+1=w1136:i32)
                        n305 = local write "liftState"(w1136) -> ()
                      }
                      frame True {
                        w1138 = 0 ("liftState")
                        n306 = global write "GlobalVI.vi" "PickingRoutine"(w1138) -> ()
                        n307 = local write "liftState"(w1138) -> ()
                      }
                    }
                  }
                  frame True {
                    n308 = global write "GlobalVI.vi" "PickingRoutine"(3 ("PickingRoutine")) -> ()
                    n309 = local write "liftState"(0 ("liftState")) -> ()
                  }
                }
              }
              frame 3 {
                # "Drives the Motor B Backwards until the switch triggers\nThen disables the motor"
                n310 = global write "GlobalVI.vi" "currentLiftState"(w1251) -> ()
                n311 = while {
                  tunnel: [w1321] -> w1250
                  tunnel: [w1330] -> w1253
                  tunnel: [w1320] -> w1249
                  stop <- w1333 stop-if-true
                  n312 = global read "GlobalVI.vi" "emergencyStop"() -> (w1326:bool)
                  n313 = xnode "Sensor 5"() -> ("B/DIO10 (Pin 31)"=w1328:bool)  [unwired: 1 in, 1 out]
                  "B/DIO10 (Pin 31) - Sensor 5\nBackwards" <- w1328
                  n314 = global read "GlobalVI.vi" "PickingRoutine"() -> (w1324:i32)
                  n315 = call "Motor_Controller.vi"("motorSelect"=enum16{"Motor A", "Motor B"}."Motor B", "direction"=enum16{"Forward", "Backward"}."Backward", "stopMotors"=FALSE) -> ("error out"=w1330:errorcluster)  [unwired: 12 in]
                  n316 = Equal?(x=w1324, y=0) -> (x = y?=w1325:bool)
                  n317 = Equal?(x=w1324, y=3) -> (x = y?=w1321:bool)
                  n318 = Or(x=w1326, y=w1325) -> (x .or. y?=w1320:bool)
                  n319 = Or(x=w1320, y=w1321) -> (x .or. y?=w1322:bool)
                  n320 = Or(x=w1328, y=w1322) -> (x .or. y?=w1333:bool)
                }
                n321 = while {
                  tunnel: TRUE ("COMM (Red)") -> [w1283]
                  stop <- w1273 stop-if-true
                  n322 = global read "GlobalVI.vi" "emergencyStop"() -> (w1274:bool)
                  n323 = feedback #7() -> (w1281:bool)  [unwired: 1 in]
                  n324 = Exclusive Or(1:w1283, 2:w1281) -> (0:w1282:bool)
                  n325 = feedback-in #7(w1282) -> ()
                  n326 = local read "liftState"() -> (w1276:i32)
                  n327 = xnode "Running LED 4"("CommG"=w1281, "CommR"=TRUE) -> ("error out"=w1278:errorcluster)  [unwired: 1 in]
                  n328 = Not Equal?(x=w1276, y=3 ("liftState")) -> (x != y?=w1275:bool)
                  n329 = Or(x=w1274, y=w1275) -> (x .or. y?=w1273:bool)
                  n330 = call "Time Delay7"("error in (no error)"=w1278, "Delay Time (s)"=0.25) -> ()  [unwired: 9 in, 1 out]
                }
                n331 = while {
                  stop <- w1266 stop-if-true
                  n332 = local read "timerCount"() -> (w1271:u32)
                  n333 = global read "GlobalVI.vi" "emergencyStop"() -> (w1270:bool)
                  n334 = Tick Count (ms)() -> (millisecond timer value=w1272:u32)
                  n335 = local read "liftState"() -> (w1268:i32)
                  n336 = Subtract(x=w1272, y=w1271) -> (x-y=w1263:u32)
                  n337 = Greater?(x=w1263, y=u32 10000) -> (0:w1264:bool)
                  n338 = local write "timeoutCounter"(w1263) -> ()
                  n339 = Not Equal?(x=w1268, y=3 ("liftState")) -> (x != y?=w1269:bool)
                  n340 = local write "timeoutError"(w1264) -> ()
                  n341 = Or(x=w1270, y=w1269) -> (x .or. y?=w1266:bool)
                }
                n342 = call "Motor_Controller.vi"("error in (no error)"=w1253, "stopMotors"=TRUE) -> ("error out"=w1252:errorcluster)  [unwired: 13 in]
                n343 = call "Time Delay 7"("error in (no error)"=w1252, "Delay Time (s)"=1.0) -> ("error out"=w1248:errorcluster)  [unwired: 9 in]
                n344 = case shown="True" w1250 {
                  tunnel: w1249 -> [w1257 _]
                  tunnel: w1248 -> [_ _]
                  frame False {
                    n345 = case shown="True" w1257 {
                      frame False {
                        n346 = local read "liftState"() -> (w1259:i32)
                        n347 = Increment(x=w1259) -> (x+1=w1258:i32)
                        n348 = local write "liftState"(w1258) -> ()
                      }
                      frame True {
                        w1260 = 0 ("liftState")
                        n349 = global write "GlobalVI.vi" "PickingRoutine"(w1260) -> ()
                        n350 = local write "liftState"(w1260) -> ()
                      }
                    }
                  }
                  frame True {
                    n351 = global write "GlobalVI.vi" "PickingRoutine"(3 ("PickingRoutine")) -> ()
                    n352 = local write "liftState"(0 ("liftState")) -> ()
                  }
                }
              }
              frame 4 {
                # "Drives the Motor A Down until the switch triggers\nThen disables the motor"
                n353 = global write "GlobalVI.vi" "currentLiftState"(w1372) -> ()
                n354 = while {
                  tunnel: TRUE ("COMM (Red)") -> [w1404]
                  stop <- w1394 stop-if-true
                  n355 = global read "GlobalVI.vi" "emergencyStop"() -> (w1395:bool)
                  n356 = feedback #8() -> (w1402:bool)  [unwired: 1 in]
                  n357 = Exclusive Or(1:w1404, 2:w1402) -> (0:w1403:bool)
                  n358 = feedback-in #8(w1403) -> ()
                  n359 = local read "liftState"() -> (w1397:i32)
                  n360 = xnode "Running LED 5"("CommG"=w1402, "CommR"=TRUE) -> ("error out"=w1399:errorcluster)  [unwired: 1 in]
                  n361 = Not Equal?(x=w1397, y=4 ("liftState")) -> (x != y?=w1396:bool)
                  n362 = Or(x=w1395, y=w1396) -> (x .or. y?=w1394:bool)
                  n363 = call "Time Delay8"("error in (no error)"=w1399, "Delay Time (s)"=0.25) -> ()  [unwired: 9 in, 1 out]
                }
                n364 = while {
                  tunnel: [w1451] -> w1374
                  tunnel: [w1444] -> w1371
                  tunnel: [w1442] -> w1370
                  stop <- w1454 stop-if-true
                  n365 = global read "GlobalVI.vi" "emergencyStop"() -> (w1447:bool)
                  n366 = xnode "Sensor 2"() -> ("B/DIO7 (Pin 25)"=w1449:bool)  [unwired: 1 in, 1 out]
                  "B/DIO7 (Pin 25) - Sensor2 - Down" <- w1449
                  n367 = global read "GlobalVI.vi" "PickingRoutine"() -> (w1445:i32)
                  n368 = call "Motor_Controller.vi"("motorSelect"=enum16{"Motor A", "Motor B"}."Motor A", "direction"=enum16{"Forward", "Backward"}."Backward", "stopMotors"=FALSE) -> ("error out"=w1451:errorcluster)  [unwired: 12 in]
                  n369 = Equal?(x=w1445, y=0) -> (x = y?=w1446:bool)
                  n370 = Equal?(x=w1445, y=3) -> (x = y?=w1444:bool)
                  n371 = Or(x=w1447, y=w1446) -> (x .or. y?=w1442:bool)
                  n372 = Or(x=w1442, y=w1444) -> (x .or. y?=w1443:bool)
                  n373 = Or(x=w1449, y=w1443) -> (x .or. y?=w1454:bool)
                }
                n374 = call "Motor_Controller.vi"("error in (no error)"=w1374, "stopMotors"=TRUE) -> ("error out"=w1373:errorcluster)  [unwired: 13 in]
                n375 = while {
                  stop <- w1387 stop-if-true
                  n376 = Tick Count (ms)() -> (millisecond timer value=w1393:u32)
                  n377 = local read "timerCount"() -> (w1392:u32)
                  n378 = global read "GlobalVI.vi" "emergencyStop"() -> (w1391:bool)
                  n379 = local read "liftState"() -> (w1389:i32)
                  n380 = Subtract(x=w1393, y=w1392) -> (x-y=w1384:u32)
                  n381 = Greater?(x=w1384, y=u32 10000) -> (0:w1385:bool)
                  n382 = Not Equal?(x=w1389, y=4 ("liftState")) -> (x != y?=w1390:bool)
                  n383 = Or(x=w1391, y=w1390) -> (x .or. y?=w1387:bool)
                  n384 = local write "timeoutCounter"(w1384) -> ()
                  n385 = local write "timeoutError"(w1385) -> ()
                }
                n386 = call "Time Delay 8"("error in (no error)"=w1373, "Delay Time (s)"=1.0) -> ("error out"=w1369:errorcluster)  [unwired: 9 in]
                n387 = case shown="True" w1371 {
                  tunnel: w1370 -> [w1378 _]
                  tunnel: w1369 -> [_ _]
                  frame False {
                    n388 = case shown="True" w1378 {
                      frame False {
                        n389 = local read "liftState"() -> (w1380:i32)
                        n390 = Increment(x=w1380) -> (x+1=w1379:i32)
                        n391 = local write "liftState"(w1379) -> ()
                      }
                      frame True {
                        w1381 = 0 ("liftState")
                        n392 = global write "GlobalVI.vi" "PickingRoutine"(w1381) -> ()
                        n393 = local write "liftState"(w1381) -> ()
                      }
                    }
                  }
                  frame True {
                    n394 = global write "GlobalVI.vi" "PickingRoutine"(3 ("PickingRoutine")) -> ()
                    n395 = local write "liftState"(0 ("liftState")) -> ()
                  }
                }
              }
              frame 5 {
                w1490 = 0 ("liftState")
                # "The lift should not run anymore"
                # "Change back to idle state and wait for next instruction"
                n396 = global write "GlobalVI.vi" "currentLiftState"(w1492) -> ()
                n397 = global write "GlobalVI.vi" "PickingRoutine"(w1490) -> ()
                n398 = local write "liftState"(w1490) -> ()
                n399 = Wait (ms)(milliseconds to wait=u32 1000) -> ()  [unwired: 1 out]
              }
            }
          }
        }
        n400 = global read "GlobalVI.vi" "emergencyStop"() -> (w57:bool)
        "timeoutError" <- FALSE ("timeoutError")
        "timeoutCounter" <- u32 0 ("timeoutCounter")
      }
    }
  }
  n401 = while {
    stop <- w1500 stop-if-true
    # "Status Updater"
    n402 = xnode "Analog input (1 sample)"() -> ("B/AI3 (Pin 9)"=→"VIN Gauge":dbl, "Emergency stop (AIPin3) (AI/AI3 (Pin 3))"=w1498:dbl)  [unwired: 1 in, 1 out]
    "Emergency stop sensor" <- w1498
    n403 = xnode "Bumper sensor"() -> ("Bumper sensor (DIO/DIO7 (Pin 7))"=w1494:bool)  [unwired: 1 in, 1 out]
    n404 = Not(x=w1494) -> (.not. x?=w1493:bool)
    "TrashCanOn" <- w1493
    n405 = global write "GlobalVI.vi" "TrashCanOn"(w1493) -> ()
    n406 = Greater Or Equal?(x=w1498, y=3.3) -> (x >= y?=w1496:bool)
    "DIO/DIO4 (Pin 4) - Emergency stop" <- w1496
    n407 = local read "timeoutError"() -> (w1502:bool)
    n408 = global read "GlobalVI.vi" "emergencyStop"() -> (w1500:bool)
    n409 = Not(x=w1502) -> (.not. x?=w1501:bool)
    n410 = global write "GlobalVI.vi" "emergencyStop"(w1496) -> ()
    n411 = global write "GlobalVI.vi" "liftStatus"(w1501) -> ()
    n412 = Wait Until Next ms Multiple(millisecond multiple=u32 250) -> ()  [unwired: 1 out]
  }
